vi "Lockin.Low Pass Filter Bank.vi"(8 "error in (no error)":errorcluster, 10 "WFms in":waveform(dbl)[](array[waveform]), 11 "Instrument.DAQ in":refnum<class "Instrument.DAQ.lvclass">) -> (0 "error out":errorcluster, 2 "Wfms out":waveform(dbl)[](array[waveform]))   [LabVIEW 2019, in "Instrument.Lockin.lvlib" / "Instrument.DAQ.lvclass"]
uses:
  Instrument.DAQ.lvclass
  <userlib>/_OpenG.lib/array/array.llb/Search 1D Array (I32)__ogtk.vi
panel:
  out "Instrument.DAQ out":refnum<class "Instrument.DAQ.lvclass">
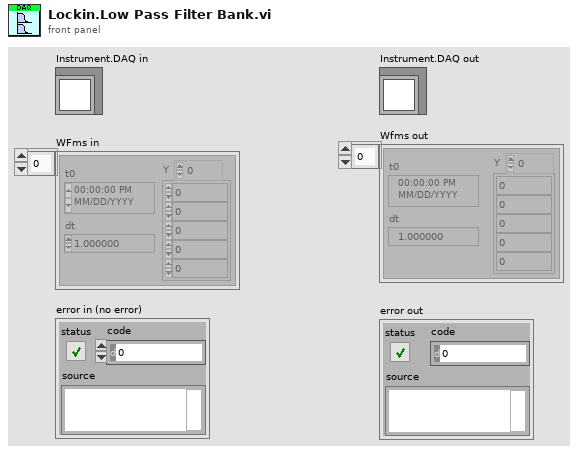
[diagram p1: front panel]
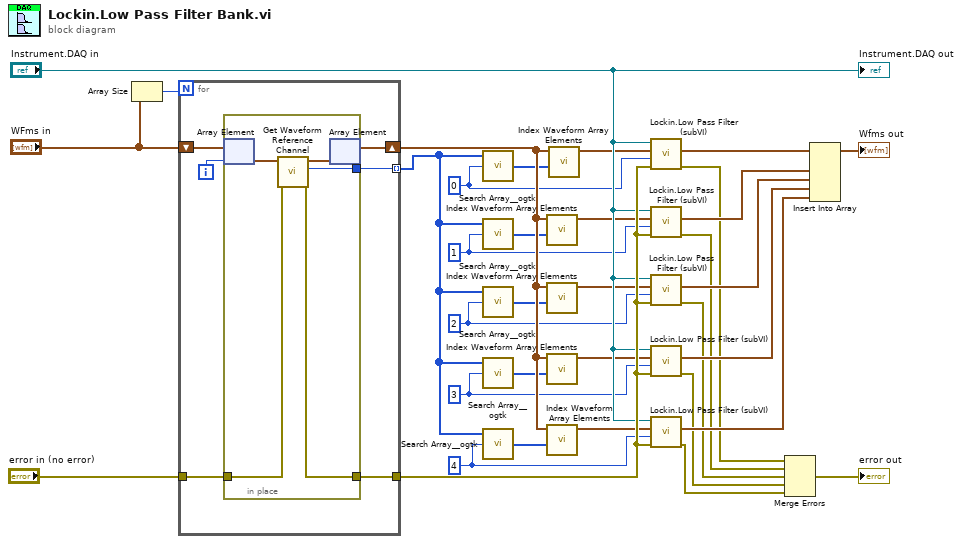
[diagram p0: block diagram]
diagram:
  w13 = 4 ("Element Data")
  w10 = 3 ("Element Data")
  w11 = 2 ("Element Data")
  w12 = 1 ("Element Data")
  w1 = 0 ("Element Data")
  n1 = Array Size(array="WFms in") -> (size(s)=w32:i32)
  n2 = for {
    N: w32 -> [_]
    shift-right: [w38] -> w27
    shift-left: "WFms in" -> [w39]
    tunnel: [w35] -> w26 mode=indexing
    tunnel: "error in (no error)" -> [w37]
    tunnel: [w36] -> w29
    i -> [w40]
    n3 = in-place {
      in-place-border: w37 -> [w43]
      in-place-border: [w42] -> w36
      in-place-border: [w41] -> w35
      n4 = in-place-array #1(w39, w40) -> (w45:waveform(dbl))
      n5 = call "Get Waveform Reference Channel.vi"("error in (no error)"=w43, "Reference in"=w45) -> ("error out"=w42:errorcluster, "Reference Channel"=w41:i32, "Reference out"=w44:waveform(dbl))  [unwired: 7 in]
      n6 = in-place-array #1(w44) -> (w38:waveform(dbl)[])  [unwired: 1 out]
    }
  }
  n7 = call-poly <userlib>:"Search Array__ogtk.vi"("Array"=w26, "Element Data"=w1) -> ("Indices of Elements"=w24:i32[])  [unwired: 7 in]
  n8 = call-poly <userlib>:"Search Array__ogtk.vi"("Array"=w26, "Element Data"=w12) -> ("Indices of Elements"=w2:i32[])  [unwired: 7 in]
  n9 = call-poly <userlib>:"Search Array__ogtk.vi"("Array"=w26, "Element Data"=w11) -> ("Indices of Elements"=w5:i32[])  [unwired: 7 in]
  n10 = call-poly <userlib>:"Search Array__ogtk.vi"("Array"=w26, "Element Data"=w10) -> ("Indices of Elements"=w6:i32[])  [unwired: 7 in]
  n11 = call-poly <userlib>:"Search Array__ogtk.vi"("Array"=w26, "Element Data"=w13) -> ("Indices of Elements"=w9:i32[])  [unwired: 7 in]
  n12 = call "Index Waveform Array Elements.vi"("Indices of Elements"=w2, "Array in"=w27) -> ("Array out"=w3:waveform(dbl)[])  [unwired: 9 in]
  n13 = call "Index Waveform Array Elements.vi"("Indices of Elements"=w5, "Array in"=w27) -> ("Array out"=w4:waveform(dbl)[])  [unwired: 9 in]
  n14 = call "Index Waveform Array Elements.vi"("Indices of Elements"=w6, "Array in"=w27) -> ("Array out"=w7:waveform(dbl)[])  [unwired: 9 in]
  n15 = call "Index Waveform Array Elements.vi"("Indices of Elements"=w9, "Array in"=w27) -> ("Array out"=w8:waveform(dbl)[])  [unwired: 9 in]
  n16 = call "Index Waveform Array Elements.vi"("Indices of Elements"=w24, "Array in"=w27) -> ("Array out"=w25:waveform(dbl)[])  [unwired: 9 in]
  n17 = call "Lockin.Low Pass Filter (subVI).vi"("error in (no error)"=w29, "Element Data"=w1, "signal in"=w25, "Lockin.DAQ in"="Instrument.DAQ in") -> ("error out"=w14:errorcluster, "signal out"=w19:waveform(dbl)[])  [unwired: 5 in, 1 out]
  n18 = call "Lockin.Low Pass Filter (subVI).vi"("error in (no error)"=w29, "Element Data"=w12, "signal in"=w3, "Lockin.DAQ in"="Instrument.DAQ in") -> ("error out"=w18:errorcluster, "signal out"=w20:waveform(dbl)[])  [unwired: 5 in, 1 out]
  n19 = call "Lockin.Low Pass Filter (subVI).vi"("error in (no error)"=w29, "Element Data"=w11, "signal in"=w4, "Lockin.DAQ in"="Instrument.DAQ in") -> ("error out"=w17:errorcluster, "signal out"=w21:waveform(dbl)[])  [unwired: 5 in, 1 out]
  n20 = call "Lockin.Low Pass Filter (subVI).vi"("error in (no error)"=w29, "Element Data"=w10, "signal in"=w7, "Lockin.DAQ in"="Instrument.DAQ in") -> ("error out"=w16:errorcluster, "signal out"=w22:waveform(dbl)[])  [unwired: 5 in, 1 out]
  n21 = call "Lockin.Low Pass Filter (subVI).vi"("error in (no error)"=w29, "Element Data"=w13, "signal in"=w8, "Lockin.DAQ in"="Instrument.DAQ in") -> ("error out"=w15:errorcluster, "signal out"=w23:waveform(dbl)[])  [unwired: 5 in, 1 out]
  n22 = Merge Errors(w14, w18, w17, w16, w15) -> (→"error out":errorcluster)
  n23 = Insert Into Array(array=w19, new element #1=w20, new element #2=w21, new element #3=w22, new element #4=w23) -> (→"Wfms out":waveform(dbl)[])  [unwired: 1 in]
  "Instrument.DAQ out" <- "Instrument.DAQ in"
